vi "Details Display Dialog.vi"(0 "Source":string caption="Quelle", 1 "Start":i32[](array[numeric]), 2 "Length":i32[](array[numeric]) caption="Länge", 5 "Details":string="Ursache des Problem\nasdfasdf\tasdfaa sdfja ;sldjf;alskdjf;a lksjdf da ist viel mehr als das Auge im ersten Moment erfassen kann ;laiwje;fliajsd;flk ajsdlkfja psoieur a;lwdjf; alksjdf;alksdjf; alksedrfap oiwejf;alkw\nwerasdf\t3425 a b c d e f g h i j k l m n o p q\nafsdfasdfasdfasdfas asdf asdf\tasdfasd", 7 "dialog type":T2 caption="Dialogtyp", 9 "Error or Warning":bool caption="Fehler oder Warnung", 11 "contname":string="OK", 12 "stopname":string="Stopp" caption="Stopname", 13 "okname":string="OK") -> (15 "stop event propagated":bool caption="Stopereignis propagieren")   [LabVIEW 2009]
uses:
  DialogTypeEnum.ctl
  ErrWarn.ctl
  eventvkey.ctl
panel:
  in  "truncated message":string="(Quelle abgeschnitten)" caption="Abgeschnittene Meldung"
  in  "truncated & CH message":string="(Quelle abgeschnitten; siehe Fenster Kontexthilfe)" caption="abgeschnittene & CH Meldungen"
  out "Source of Error":string caption="Fehlerquelle"
  out "scrollbar text":string caption="Rollbalken-Text"
  in  "Test for size":string caption="Test auf Größe"
  out "text":string caption="Text"
  out "Error or Warning Glyph":T1=TRUE caption="Fehler- oder Warnungssymbol"
  in  "OK":bool
  in  "Stop":bool caption="Stopp"
  in  "Continue":bool caption="OK"
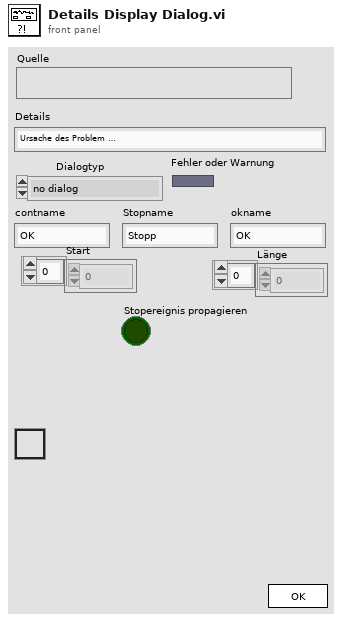
[diagram p1: front panel]
types:
  T1 = typedef "ErrWarn.ctl" = bool
  T2 = typedef "DialogTypeEnum.ctl" = enum16{"no dialog", "OK message", "continue or stop message", "auto error handling dialog", "OK message + warnings", "continue/stop + warnings"}
  T3 = typedef "LVRectTypeDef.ctl" = cluster{"left":i16, "top":i16, "right":i16, "bottom":i16}
  T4 = cluster{"Control":bool, "Shift":bool, "Key":string}
  T5 = typedef "eventvkey.ctl" = enum16{"ASCII", "Enter", "Shift", "Ctrl", "Alt", "Cmd", "Opt", "Caps", "NumLock", "Clear", "Break", "Up", "Down", "Left", "Right", "Insert", "Delete", "Home", "End", "PageUp", "PageDown", "Escape", "Help", "Pause", "ScrollLock", "F1", "F2", "F3", "F4", "F5", "F6", "F7", "F8", "F9", "F10", "F11", "F12", "Two Byte Char"}
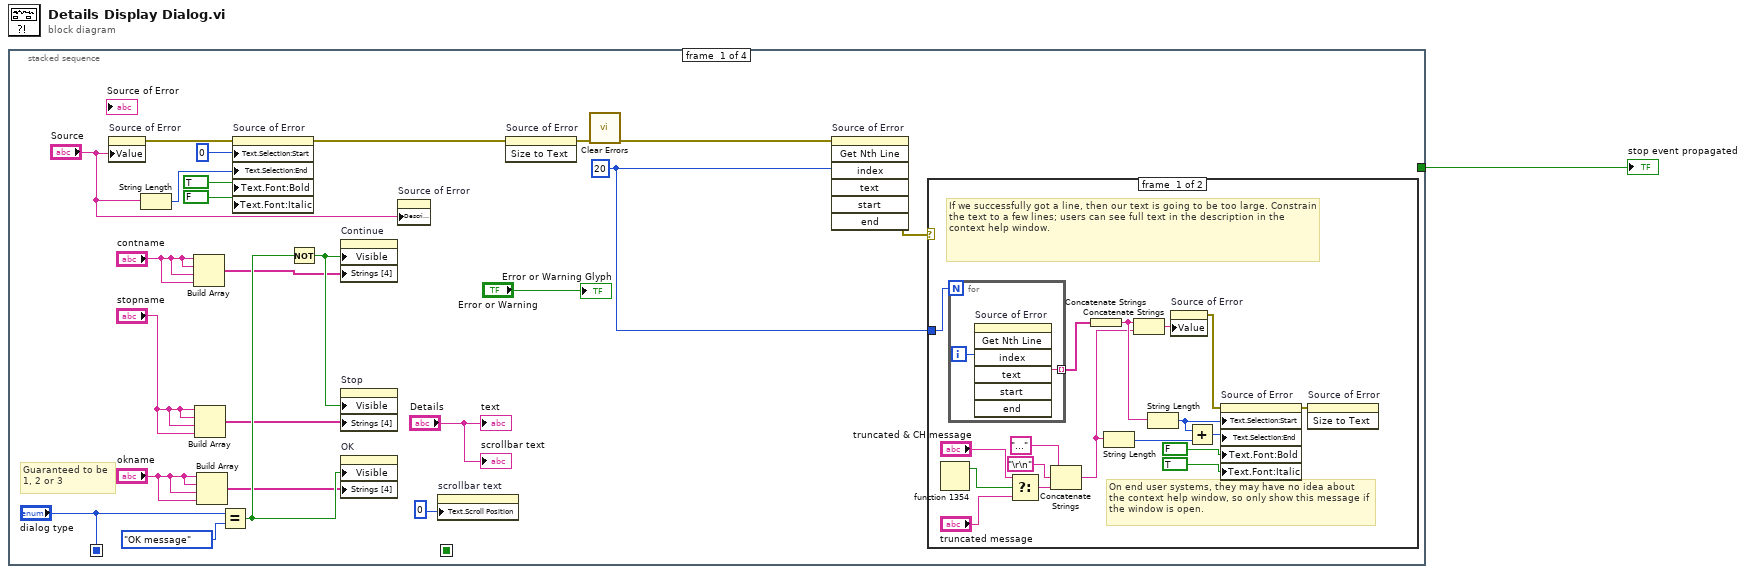
[diagram p0: block diagram]
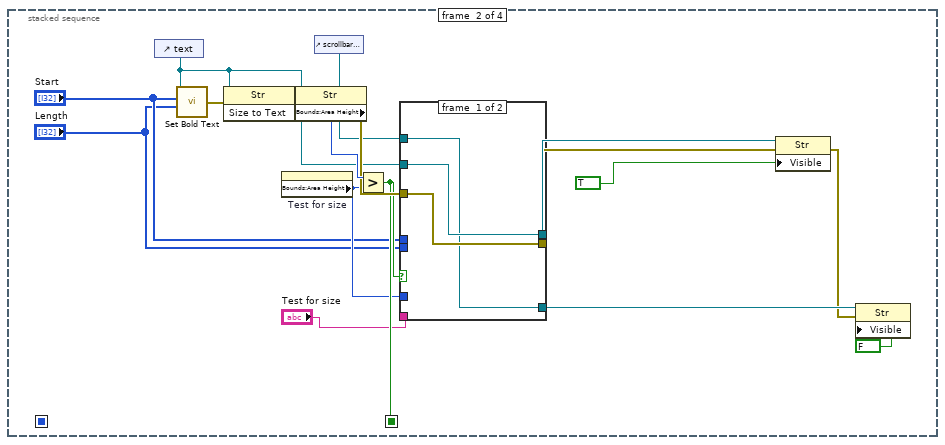
[diagram p3: hidden frame]
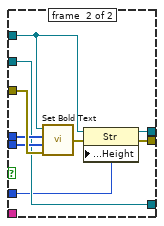
[diagram p4: hidden frame]
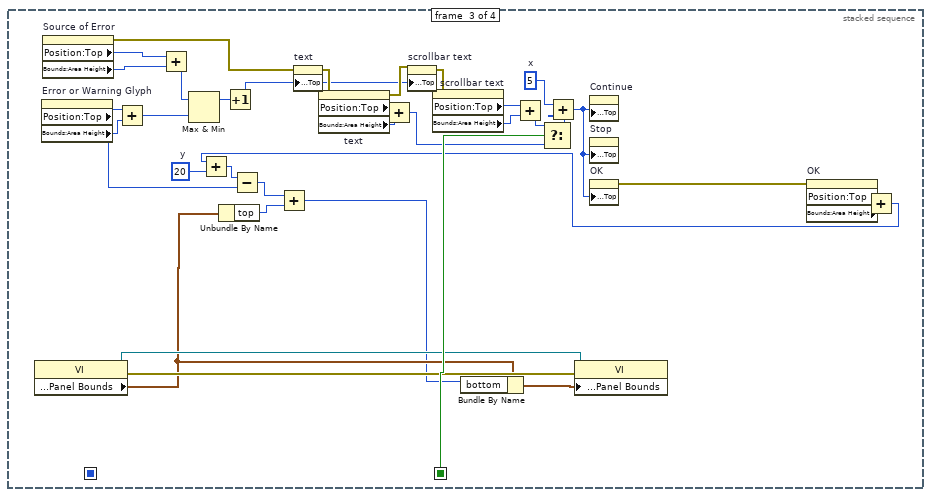
[diagram p5: hidden frame]
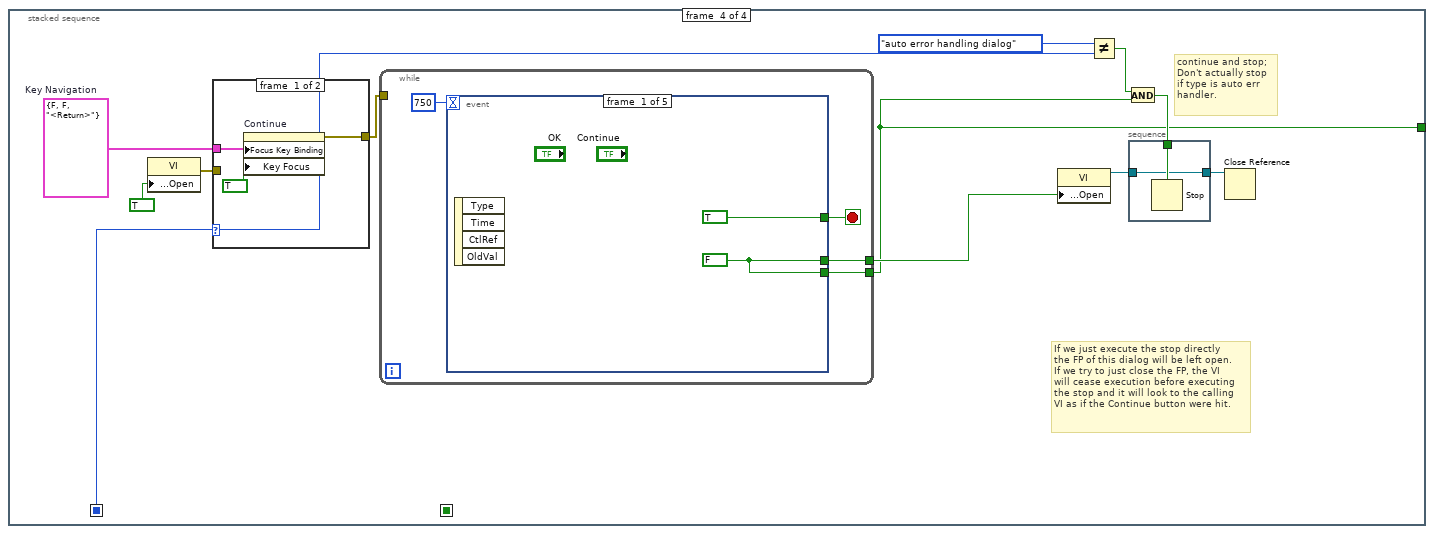
[diagram p6: hidden frame]
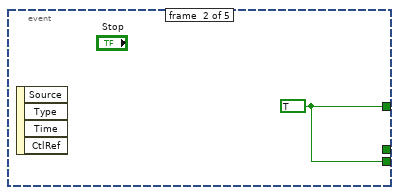
[diagram p7: hidden frame]
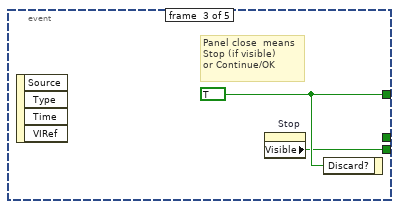
[diagram p8: hidden frame]
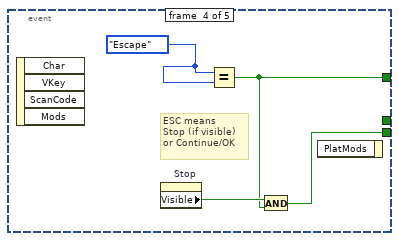
[diagram p9: hidden frame]
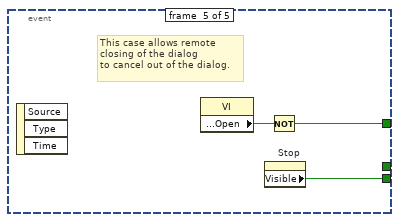
[diagram p10: hidden frame]
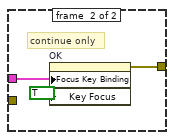
[diagram p11: hidden frame]
diagram:
  n1 = stacked-sequence {
    seq-local: ["dialog type" _ _ _] -> [_ _ _ w112]
    seq-local: [_ w54 _ _] -> [_ _ w109 _]
    tunnel: [_ _ _ w110] -> w1
    frame #0 {
      w9 = u32 20 ("index")
      # "Guaranteed to be\n1, 2 or 3"
      n2 = property on="Source of Error" class="Str"("Value"="Source") -> (error out=w8:errorcluster)  [unwired: 2 in, 1 out]
      n3 = String Length(string="Source") -> (length=w4:i32)
      n4 = Build Array("contname", "contname", "contname", "contname") -> (w18:string[])
      n5 = Build Array("stopname", "stopname", "stopname", "stopname") -> (w17:string[])
      n6 = Build Array("okname", "okname", "okname", "okname") -> (w16:string[])
      n7 = Equal?(x="dialog type", y=DialogTypeEnum."OK message" ("dialog type")) -> (x = y?=w22:bool)
      n8 = property on="Source of Error" class="Str"(error in=w8, "Text.Selection:Start"=u32 0, "Text.Selection:End"=w4, "Text.Font:Bold"=TRUE, "Text.Font:Italic"=FALSE) -> (error out=w7:errorcluster)  [unwired: 1 in, 1 out]
      n9 = Not(x=w22) -> (.not. x?=w21:bool)
      n10 = property on="Continue" class="Boolean"("Visible"=w21, "Strings [4]"=w18) -> ()  [unwired: 2 in, 2 out]
      n11 = property on="Stop" class="Boolean"("Visible"=w21, "Strings [4]"=w17) -> ()  [unwired: 2 in, 2 out]
      n12 = property on="OK" class="Boolean"("Visible"=w22, "Strings [4]"=w16) -> ()  [unwired: 2 in, 2 out]
      n13 = property on="Source of Error" class="Str"("Description"="Source") -> ()  [unwired: 2 in, 2 out]
      n14 = property on="scrollbar text" class="String"("Text.Scroll Position"=0) -> ()  [unwired: 2 in, 2 out]
      n15 = invoke on="Source of Error" class="Str" method="Size to Text"(error in=w7) -> (error out=w12:errorcluster)  [unwired: 2 in, 2 out]
      n16 = call "Clear Errors.vi"("error in (no error)"=w12) -> ("error out"=w11:errorcluster)  [unwired: 6 in]
      n17 = invoke on="Source of Error" class="Str" method="Get Nth Line"(error in=w11, "index"=w9) -> (error out=w10:errorcluster)  [unwired: 5 in, 6 out]
      n18 = case shown="No Error" w10 {
        tunnel: w9 -> [w43 _]
        frame #0 {
          # "On end user systems, they may have no idea about\nthe context help window, so only show this message if\nthe window is open."
          # "If we successfully got a line, then our text is going to be too large. Constrain the text to a few lines; users can see full text in the description in the context help window."
          n19 = fn#1354() -> (1:w33:bool)  [unwired: 1 out]
          n20 = for {
            N: w43 -> [_]
            tunnel: [w44] -> w41 mode=indexing
            i -> [w45]
            n21 = invoke on="Source of Error" class="Str" method="Get Nth Line"("index"=w45) -> ("text"=w44:string)  [unwired: 6 in, 6 out]
          }
          n22 = Select(t="truncated & CH message", s=w33, f="truncated message") -> (s? t:f=w30:string)
          n23 = Concatenate Strings("..." ("string"), "\r\n", w30) -> (w27:string)
          n24 = Concatenate Strings(w41) -> (w40:string)
          n25 = String Length(string=w27) -> (length=w32:i32)
          n26 = Concatenate Strings(w40, w27) -> (w42:string)
          n27 = String Length(string=w40) -> (length=w35:i32)
          n28 = property on="Source of Error" class="Str"("Value"=w42) -> (error out=w37:errorcluster)  [unwired: 2 in, 1 out]
          n29 = Add(x=w35, y=w32) -> (x+y=w34:i32)
          n30 = property on="Source of Error" class="Str"(error in=w37, "Text.Selection:Start"=w35, "Text.Selection:End"=w34, "Text.Font:Bold"=FALSE, "Text.Font:Italic"=TRUE) -> (error out=w36:errorcluster)  [unwired: 1 in, 1 out]
          n31 = invoke on="Source of Error" class="Str" method="Size to Text"(error in=w36) -> ()  [unwired: 2 in, 3 out]
        }
        frame #1 {
          # "An error at this point means that there is no line to fetch. That's good. We do not want the text getting too large."
        }
      }
      "Error or Warning Glyph" <- "Error or Warning"
      "scrollbar text" <- "Details"
      "text" <- "Details"
    }
    frame #1 {
      n32 = control-ref of="text"() -> (w49:refnum<vi>)
      n33 = call "Set Bold Text.vi"("Length"="Length", "Start"="Start", "text"=w49) -> ("error out"=w52:errorcluster)  [unwired: 3 in]
      n34 = invoke class="Str" method="Size to Text"(reference=w49, error in=w52) -> (error out=w53:errorcluster)  [unwired: 1 in, 2 out]
      n35 = property on="Test for size" class="String"() -> ("Bounds:Area Height"=w51:u32)  [unwired: 2 in, 2 out]
      n36 = property class="Str"(reference=w49, error in=w53) -> (error out=w61:errorcluster, "Bounds:Area Height"=w62:u32)  [unwired: 1 out]
      n37 = control-ref of="scrollbar text"() -> (w57:refnum<vi>)
      n38 = Greater?(x=w62, y=w51) -> (0:w54:bool)
      n39 = case shown="True" w54 {
        tunnel: w61 -> [w65 w74]
        tunnel: "Start" -> [_ w73]
        tunnel: "Length" -> [_ w72]
        tunnel: [w65 w69] -> w50
        tunnel: w49 -> [w64 w71]
        tunnel: [w64 w66] -> w59
        tunnel: [w63 w71] -> w58
        tunnel: w57 -> [w63 w67]
        tunnel: w51 -> [_ w70]
        tunnel: "Test for size" -> [_ _]
        frame #0 {
        }
        frame #1 {
          n40 = call "Set Bold Text.vi"("error in"=w74, "Length"=w72, "Start"=w73, "text"=w67) -> ("error out"=w68:errorcluster)  [unwired: 2 in]
          n41 = property class="Str"(reference=w67, error in=w68, "Text Size:Height"=w70) -> (reference out=w66:refnum<vi>, error out=w69:errorcluster)
        }
      }
      n42 = property class="Str"(reference=w59, error in=w50, "Visible"=TRUE ("Defer Panel Updates")) -> (error out=w55:errorcluster)  [unwired: 1 out]
      n43 = property class="Str"(reference=w58, error in=w55, "Visible"=FALSE ("Defer Panel Updates")) -> ()  [unwired: 2 out]
    }
    frame #2 {
      w95 = u32 20  # y
      w100 = u32 5  # x
      n44 = property class="VI"() -> (reference out=w92:refnum<vi>, error out=w93:errorcluster, "Front Panel Window:Panel Bounds"=w89:T3)  [unwired: 2 in]
      n45 = property on="Error or Warning Glyph" class="Boolean"() -> ("Position:Top"=w90:i32, "Bounds:Area Height"=w106:u32)  [unwired: 2 in, 2 out]
      n46 = property on="Source of Error" class="String"() -> (error out=w75:errorcluster, "Position:Top"=w77:i32, "Bounds:Area Height"=w76:u32)  [unwired: 2 in, 1 out]
      n47 = Add(x=w90, y=w106) -> (x+y=w107:u32)
      n48 = Add(x=w77, y=w76) -> (x+y=w108:u32)
      n49 = Max & Min(x=w108, y=w107) -> (max(x,y)=w105:u32)  [unwired: 1 out]
      n50 = Unbundle By Name(w89) -> ("top"=w87:i16)
      n51 = Increment(x=w105) -> (x+1=w83:u32)
      n52 = property on="text" class="Str"(error in=w75, "Position:Top"=w83) -> (error out=w85:errorcluster)  [unwired: 1 in, 1 out]
      n53 = property on="text" class="Str"(error in=w85) -> (error out=w84:errorcluster, "Position:Top"=w82:i32, "Bounds:Area Height"=w81:u32)  [unwired: 1 in, 1 out]
      n54 = Add(x=w82, y=w81) -> (x+y=w79:u32)
      n55 = property on="scrollbar text" class="String"(error in=w84, "Position:Top"=w83) -> (error out=w104:errorcluster)  [unwired: 1 in, 1 out]
      n56 = property on="scrollbar text" class="String"(error in=w104) -> ("Position:Top"=w103:i32, "Bounds:Area Height"=w102:u32)  [unwired: 1 in, 2 out]
      n57 = Add(x=w103, y=w102) -> (x+y=w80:u32)
      n58 = Select(t=w80, s=w109, f=w79) -> (s? t:f=w78:u32)
      n59 = Add(x=w100, y=w78) -> (x+y=w101:u32)
      n60 = property on="Continue" class="Boolean"("Position:Top"=w101) -> ()  [unwired: 2 in, 2 out]
      n61 = property on="Stop" class="Bool"("Position:Top"=w101) -> ()  [unwired: 2 in, 2 out]
      n62 = property on="OK" class="Bool"("Position:Top"=w101) -> (error out=w99:errorcluster)  [unwired: 2 in, 1 out]
      n63 = property on="OK" class="Bool"(error in=w99) -> ("Position:Top"=w97:i32, "Bounds:Area Height"=w98:u32)  [unwired: 1 in, 2 out]
      n64 = Add(x=w97, y=w98) -> (x+y=w96:u32)
      n65 = Add(x=w96, y=w95) -> (x+y=w91:u32)
      n66 = Subtract(x=w91, y=w90) -> (x-y=w88:u32)
      n67 = Add(x=w88, y=w87) -> (x+y=w86:u32)
      n68 = Bundle By Name(cluster=w89, "bottom"=w86) -> (w94:T3)
      n69 = property class="VI"(reference=w92, error in=w93, "Front Panel Window:Panel Bounds"=w94) -> ()  [unwired: 2 out]
    }
    frame #3 {
      w121 = T4 {"Control"=FALSE, "Shift"=FALSE, "Key"="<Return>"}  # Key Navigation
      # "If we just execute the stop directly\nthe FP of this dialog will be left open.\nIf we try to just close the FP, the VI\nwill cease execution before executing\nthe stop and it will look to the calling\nVI as if the Continue button were hit."
      # "continue and stop;\nDon't actually stop\nif type is auto err\nhandler."
      n70 = property class="VI"("Front Panel Window:Open"=TRUE) -> (error out=w120:errorcluster)  [unwired: 2 in, 1 out]
      n71 = case shown="\"continue or stop message\", Default" w112 {
        tunnel: w121 -> [w142 w145]
        tunnel: w120 -> [_ _]
        tunnel: [w140 w143] -> w118
        frame #0 {
          n72 = property on="Continue" class="Boolean"("Focus Key Binding"=w142, "Key Focus"=TRUE) -> (error out=w140:errorcluster)  [unwired: 2 in, 1 out]
        }
        frame #1 {
          # "continue only"
          n73 = property on="OK" class="Boolean"("Focus Key Binding"=w145, "Key Focus"=TRUE) -> (error out=w143:errorcluster)  [unwired: 2 in, 1 out]
        }
      }
      n74 = while {
        tunnel: w118 -> [_]
        tunnel: [w126] -> w110
        tunnel: [w125] -> w111
        stop <- w127 stop-if-true
        n75 = event shown="[3] Key Down?" {
          selector: _ -> [_ _ _ _ _]
          dyn-events: _ -> [_ _ _ _ _]
          timeout: 750 -> [_ _ _ _ _]
          tunnel: [TRUE ("Stop") w130 w132 w134 w137] -> w127
          tunnel: [w129 w130 w131 w135 w139] -> w126
          tunnel: [w129 _ _ _ _] -> w125
          event #0 {
            w129 = FALSE ("Stop")
            n76 = event-data() -> ()  [unwired: 1 in, 4 out]
          }
          event #1 {
            w130 = TRUE
            n77 = event-data() -> ()  [unwired: 1 in, 4 out]
          }
          event #2 {
            w132 = TRUE ("Discard?")
            # "Panel close  means\nStop (if visible)\nor Continue/OK"
            n78 = event-data() -> ()  [unwired: 1 in, 4 out]
            n79 = property on="Stop" class="Boolean"() -> ("Visible"=w131:bool)  [unwired: 2 in, 2 out]
            n80 = event-data("Discard?"=w132) -> ()  [unwired: 1 in, 1 out]
          }
          event #3 {
            w133 = eventvkey."Escape" ("x")
            # "ESC means\nStop (if visible)\nor Continue/OK"
            n81 = event-data() -> ()  [unwired: 1 in, 4 out]
            n82 = property on="Stop" class="Boolean"() -> ("Visible"=w136:bool)  [unwired: 2 in, 2 out]
            n83 = Equal?(x=w133, y=w133) -> (x = y?=w134:bool)
            n84 = And(x=w136, y=w134) -> (x .and. y?=w135:bool)
            n85 = event-data() -> ()  [unwired: 2 in, 1 out]
          }
          event #4 {
            # "This case allows remote\nclosing of the dialog\nto cancel out of the dialog."
            n86 = event-data() -> ()  [unwired: 1 in, 3 out]
            n87 = property class="VI"() -> ("Front Panel Window:Open"=w138:bool)  [unwired: 2 in, 2 out]
            n88 = property on="Stop" class="Boolean"() -> ("Visible"=w139:bool)  [unwired: 2 in, 2 out]
            n89 = Not(x=w138) -> (.not. x?=w137:bool)
          }
        }
      }
      n90 = property class="VI"("Front Panel Window:Open"=w111) -> (reference out=w114:refnum<vi>)  [unwired: 2 in, 1 out]
      n91 = Not Equal?(x=DialogTypeEnum."auto error handling dialog" ("dialog type"), y=w112) -> (x != y?=w117:bool)
      n92 = And(x=w117, y=w110) -> (x .and. y?=w116:bool)
      n93 = stacked-sequence {
        tunnel: w114 -> [w122]
        tunnel: w116 -> [w123]
        tunnel: [w122] -> w115
        frame #0 {
          n94 = Stop(stop? (T)=w123) -> ()
        }
      }
      n95 = Close Reference(reference=w115) -> ()  [unwired: 1 in, 1 out]
    }
  }
  "stop event propagated" <- w1
